vi "RealWorldToPixelCoordinates.vi"(7 "error in (no error)":errorcluster, 9 "Real World Points":dbl[][](array[numeric]), 10 "Calibration 2":T1={"Pixel Width (X)"=1.0, "Pixel Height (Y)"=1.0}) -> (0 "error out":errorcluster, 3 "Pixels":dbl[][](array[numeric]))   [LabVIEW 2017, in "ImageAcquisitionLibrary.lvlib"]
uses:
  ImageAcquisitionLibrary.lvlib
  Settings/Calibration.ctl
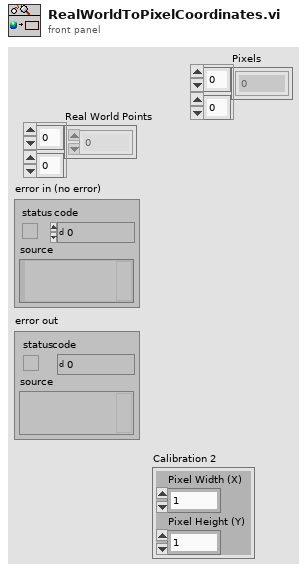
[diagram p1: front panel]
types:
  T1 = typedef "ImageAcquisitionLibrary.lvlib/Calibration.ctl" = cluster{"Pixel Width (X)":dbl, "Pixel Height (Y)":dbl}
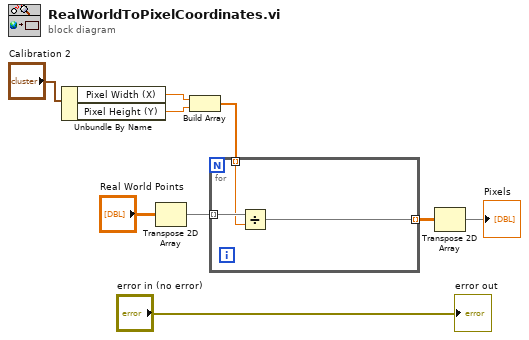
[diagram p0: block diagram]
diagram:
  n1 = Unbundle By Name("Calibration 2") -> ("Pixel Width (X)"=w9:dbl, "Pixel Height (Y)"=w8:dbl)
  n2 = Transpose 2D Array(2D array="Real World Points") -> (transposed array=w3:dbl[][])
  n3 = Build Array(w9, w8) -> (w7:dbl[])
  n4 = for {
    tunnel: w3 -> [w11] mode=indexing
    tunnel: w7 -> [w10] mode=indexing
    tunnel: [w12] -> w5 mode=indexing
    n5 = Divide(x=w11, y=w10) -> (x/y=w12:dbl[])
  }
  n6 = Transpose 2D Array(2D array=w5) -> (transposed array=→"Pixels":dbl[][])
  "error out" <- "error in (no error)"
